vi "Remove Header.vi"(8 "error in":errorcluster, 10 "header":string, 11 "http-client in":refnum<class "http-client.lvclass">) -> (0 "error out":errorcluster, 3 "http-client out":refnum<class "http-client.lvclass">)   [LabVIEW 2020, in "REST Client.lvlib" / "http-client.lvclass"]
uses:
  http-client.lvclass
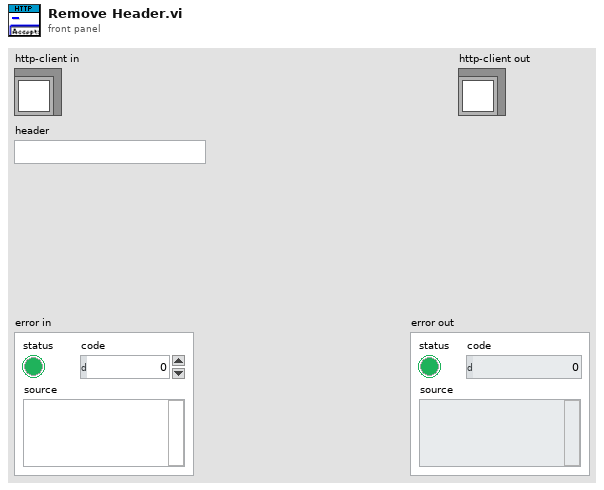
[diagram p1: front panel]
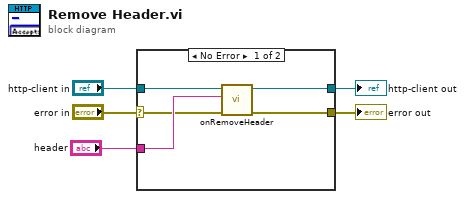
[diagram p0: block diagram]
diagram:
  n1 = case shown="No Error" "error in" {
    selector: "error in" -> [w8 w12]
    tunnel: [w7 w12] -> w4
    tunnel: [w6 w11] -> w2
    tunnel: "http-client in" -> [w10 w11]
    tunnel: "header" -> [w9 _]
    frame No Error {
      n2 = call-dynamic "onRemoveHeader.vi"("error in"=w8, "header"=w9, "http-client in"=w10) -> ("error out"=w7:errorcluster, "http-client out"=w6:refnum<class "http-client.lvclass">)  [unwired: 7 in]
    }
    frame Error {
    }
  }
  "error out" <- w4
  "http-client out" <- w2
